vi "WebCAM_Init.vi"(8 "error in (no error)":errorcluster, 10 "PictureBox":refnum<k24>, 11 "Window Title":string="Title") -> (0 "error out":errorcluster)   [LabVIEW 2020]
uses:
  System.Windows.Forms
  avicap32.dll
  user32.dll
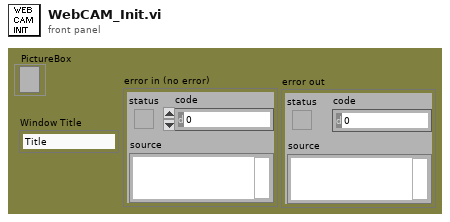
[diagram p1: front panel]
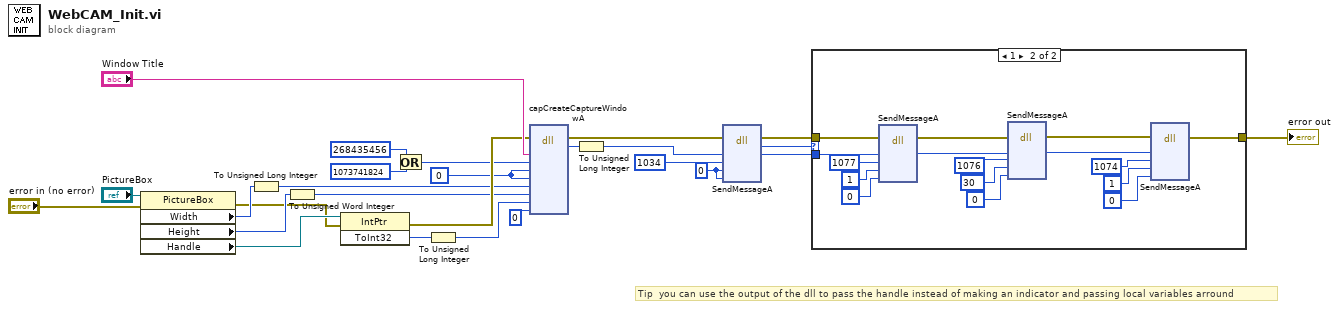
[diagram p0: block diagram]
diagram:
  w8 = u32 0 ("wParam")
  w11 = u32 0 ("y")
  # "Tip  you can use the output of the dll to pass the handle instead of making an indicator and passing local variables arround"
  n1 = property class="PictureBox"(reference="PictureBox", error in="error in (no error)") -> (error out=w20:errorcluster, "Width"=w22:i32, "Height"=w23:i32, "Handle"=w21:refnum<k24>)  [unwired: 1 out]
  n2 = To Unsigned Long Integer(number=w22) -> (unsigned 32bit integer=w19:u32)
  n3 = To Unsigned Word Integer(number=w23) -> (unsigned 16bit integer=w17:u16)
  n4 = invoke class="IntPtr" method="ToInt32"(reference=w21, error in=w20) -> (error out=w24:errorcluster, "ToInt32"=w12:i32)  [unwired: 1 in, 1 out]
  n5 = Or(x=u32 268435456, y=u32 1073741824) -> (x .or. y?=w15:u32)
  n6 = To Unsigned Long Integer(number=w12) -> (unsigned 32bit integer=w18:u32)
  n7 = dll-call lib="avicap32.dll" fn="capCreateCaptureWindowA"(error in=w24, "lpszWindowName"="Window Title", "dwStyle"=w15, "x"=w11, "y"=w11, "nWidth"=w19, "nHeight"=w17, "hwnd"=w18, "nID"=u32 0) -> (error out=w3:errorcluster, "return type"=w5:i32)  [unwired: 10 in, 1 out]
  n8 = To Unsigned Long Integer(number=w5) -> (unsigned 32bit integer=w6:u32)
  n9 = dll-call lib="user32.dll" fn="SendMessageA"(error in=w3, "hwnd"=w6, "msg"=u32 1034, "wParam"=w8, "lparam"=w8) -> (error out=w2:errorcluster, "return type"=w7:u32, "hwnd"=w4:u32)  [unwired: 5 in, 1 out]
  n10 = case shown="1" w7 {
    tunnel: w4 -> [_ w43]
    tunnel: w2 -> [w27 w29]
    tunnel: [w27 w28] -> w25
    frame 0, Default {
    }
    frame 1 {
      n11 = dll-call lib="user32.dll" fn="SendMessageA"(error in=w29, "hwnd"=w43, "msg"=u32 1077, "wParam"=u32 1 ("msg"), "lparam"=u32 0 ("msg")) -> (error out=w36:errorcluster, "hwnd"=w35:u32)  [unwired: 6 in, 1 out]
      n12 = dll-call lib="user32.dll" fn="SendMessageA"(error in=w36, "hwnd"=w35, "msg"=u32 1076, "wParam"=u32 30 ("msg"), "lparam"=u32 0 ("msg")) -> (error out=w31:errorcluster, "hwnd"=w30:u32)  [unwired: 6 in, 1 out]
      n13 = dll-call lib="user32.dll" fn="SendMessageA"(error in=w31, "hwnd"=w30, "msg"=u32 1074, "wParam"=u32 1 ("msg"), "lparam"=u32 0 ("msg")) -> (error out=w28:errorcluster)  [unwired: 7 in, 1 out]
    }
  }
  "error out" <- w25
